vi "Loop Pause Check.vi"(0 "Pause":T1, 1 "Stop":bool) -> (2 "Pause":bool, 3 "State":string, 4 "ABORT":bool)   [LabVIEW 2019]
doc: "Checks the pause and stop buttons in a loop.\nScott Hannahs, FBNML, Jan 1992"
uses:
  Sub Controls/Pause Switch.ctl
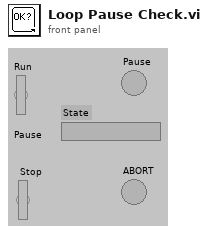
[diagram p1: front panel]
types:
  T1 = typedef "Pause Switch.ctl" = bool
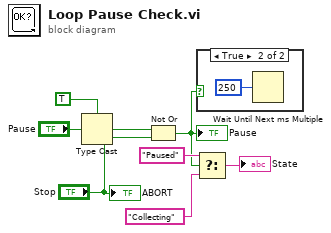
[diagram p0: block diagram]
diagram:
  n1 = Type Cast(type=TRUE, x="Pause") -> (*(type *) &x=w3:bool)
  n2 = Not Or(1:"Stop", 2:w3) -> (0:w5:bool)
  "Pause" <- w5
  n3 = case shown="True" w5 {
    frame False {
    }
    frame True {
      n4 = Wait Until Next ms Multiple(millisecond multiple=u32 250) -> ()  [unwired: 1 out]
    }
  }
  n5 = Select(t="Paused", s=w5, f="Collecting") -> (s? t:f=→"State":string)
  "ABORT" <- "Stop"
